vi "Open Device.vi"(7 "Device Type":string, 8 "error in (no error)":errorcluster, 10 "Device Identifier":string, 11 "Mercury Reference In":T1) -> (0 "error out":errorcluster, 3 "Mercury Reference Out":T1)   [LabVIEW 2014, in "Mercury iXX.lvlib" / "System.lvlib"]
doc: "Opens a reference to a device within the current Mercury instrument you are connected to.\n\nOpen System must be called before this function."
uses:
  System.lvlib
  Controls/Mercury Reference.ctl
  Controls/Comms Transport Layer.ctl
  Private/Controls/Query Dynamic Reference.ctl
  Mercury iXX.lvlib
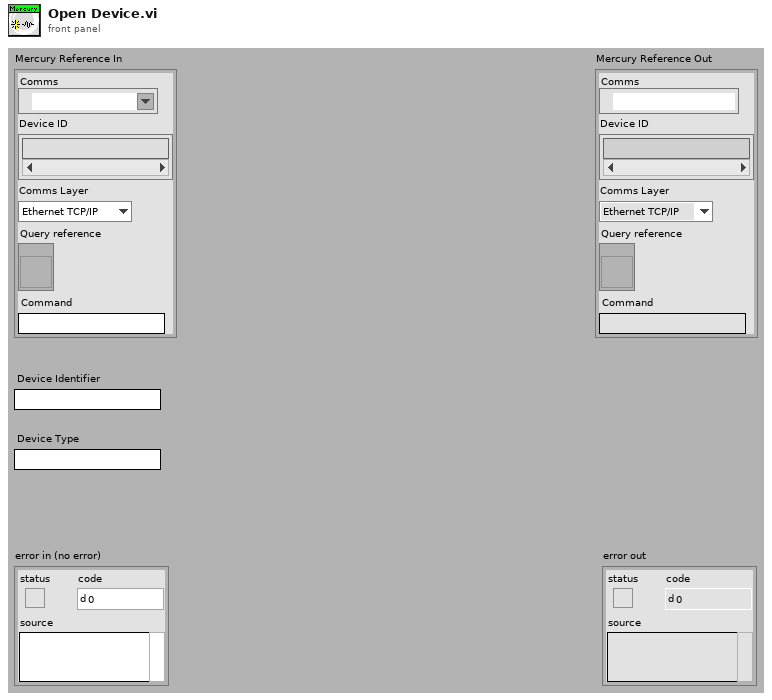
[diagram p1: front panel]
types:
  T1 = typedef "Mercury iXX.lvlib/Mercury Reference.ctl" = cluster{"Comms":refnum<visa-resource-name>, "Device ID":string[], "Comms Layer":T2, "Command":string, "Query reference":T3}
  T2 = typedef "Mercury iXX.lvlib/Comms Transport Layer.ctl" = enum16{"Ethernet TCP/IP", "USB", "ISOBus - RS-232", "GPIB"}
  T3 = typedef "Mercury iXX.lvlib/Query Dynamic Reference.ctl" = refnum<vi>
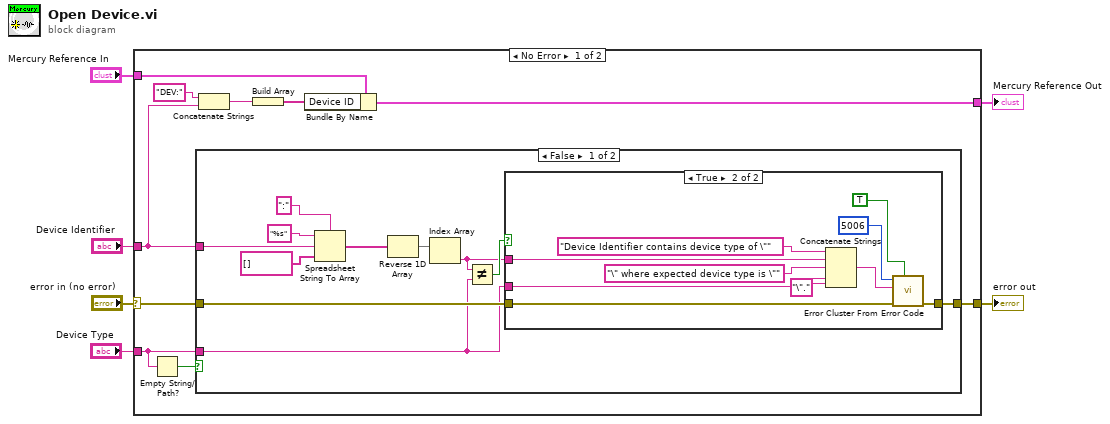
[diagram p0: block diagram]
diagram:
  n1 = case shown="No Error" "error in (no error)" {
    selector: "error in (no error)" -> [w9 w41]
    tunnel: "Mercury Reference In" -> [w16 w40]
    tunnel: [w15 w40] -> w5
    tunnel: [w8 w41] -> w3
    tunnel: "Device Identifier" -> [w11 _]
    tunnel: "Device Type" -> [w7 _]
    frame No Error {
      n2 = Empty String/Path?(string/path=w7) -> (empty?=w10:bool)
      n3 = case shown="False" w10 {
        tunnel: w11 -> [w27 _]
        tunnel: [w19 w39] -> w8
        tunnel: w9 -> [w20 w39]
        tunnel: w7 -> [w18 _]
        frame False {
          n4 = Spreadsheet String To Array(delimiter (Tab)=":", format string="%s", spreadsheet string=w27, array type (2D Dbl)=string[] []) -> (array=w23:string[])
          n5 = Reverse 1D Array(array=w23) -> (reversed array=w22:string[])
          n6 = Index Array(array=w22) -> (element=w17:string)  [unwired: 1 in]
          n7 = Not Equal?(x=w17, y=w18) -> (x != y?=w21:bool)
          n8 = case shown="True" w21 {
            tunnel: [w28 w37] -> w19
            tunnel: w20 -> [w28 w38]
            tunnel: w18 -> [_ w30]
            tunnel: w17 -> [_ w32]
            frame False {
            }
            frame True {
              n9 = Concatenate Strings("Device Identifier contains device type of \"" ("error message (\"\")"), w32, "\" where expected device type is \"" ("string"), w30, "\"." ("string")) -> (w33:string)
              n10 = call <vilib>:"Error Cluster From Error Code.vi"("show call chain? (False)"=TRUE, "error in (no error)"=w38, "error message (\"\")"=w33, "error code (0)"=5006) -> ("error out"=w37:errorcluster)  [unwired: 5 out]
            }
          }
        }
        frame True {
        }
      }
      n11 = Concatenate Strings("DEV:" ("element"), w11) -> (w13:string)
      n12 = Build Array(w13) -> (w14:string[])
      n13 = Bundle By Name(cluster=w16, "Device ID"=w14) -> (w15:T1)
    }
    frame Error {
    }
  }
  "Mercury Reference Out" <- w5
  "error out" <- w3
